vi "q2DCM (SubVI).vi"(11 "Quaternion":sgl[](array[numeric])=[0.0, 0.0, 0.0, 1.0]) -> (1 "DCM line 3":sgl[](array[numeric]), 2 "DCM line 2":sgl[](array[numeric]), 3 "DCM line 1":sgl[](array[numeric]))   [LabVIEW 2017]
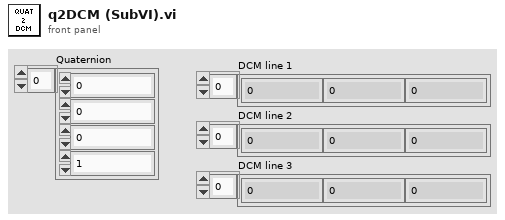
[diagram p1: front panel]
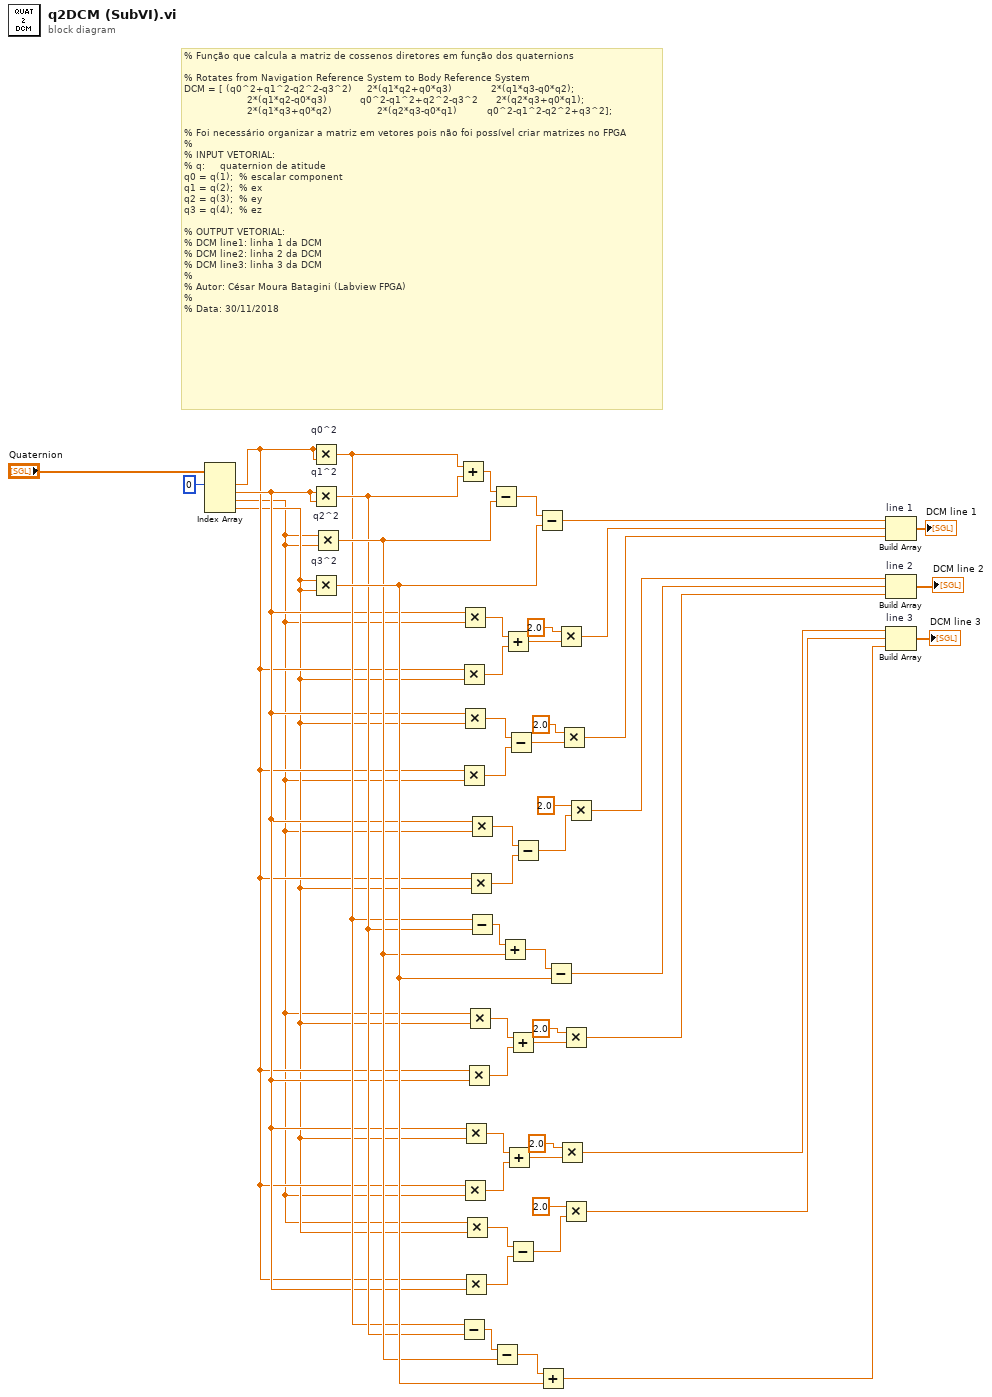
[diagram p0: block diagram]
diagram:
  # "% Função que calcula a matriz de cossenos diretores em função dos quaternions\n\n% Rotates from Navigation Reference System to Body Reference System\nDCM = [ (q0^2+q1^2-q2^2-q3^2)     2*(q1*q2+q0*q3)             2*(q1*q3-q0*q2);\n                     2*(q1*q2-q0*q3)           q0^2-q1^2+q2^2-q3^2      2*(q2*q3+q0*q1);\n                     2*(q1*q3+q0*q2)               2*(q2*q3-q0*q1)          q0^2-q1^2-q2^2+q3^2];\n\n% Foi necessário organizar a matriz em vetores pois não foi possível criar matrizes no FPGA\n%\n% INPUT VETORIAL: \n% q:     quaternion de atitude   \nq0 = q(1);  % escalar component\nq1 = q(2);  % ex\nq2 = q(3);  % ey\nq3 = q(4);  % ez\n\n% OUTPUT VETORIAL:\n% DCM line1: linha 1 da DCM\n% DCM line2: linha 2 da DCM\n% DCM line3: linha 3 da DCM\n%\n% Autor: César Moura Batagini (Labview FPGA)\n%             \n% Data: 30/11/2018"
  n1 = Index Array(array="Quaternion", index #1=0 ("index")) -> (element #1=w47:sgl, element #2=w48:sgl, element #3=w45:sgl, element #4=w46:sgl)  [unwired: 3 in]
  n2 = Multiply "q0^2"(x=w47, y=w47) -> (x*y=w49:sgl)
  n3 = Multiply "q1^2"(x=w48, y=w48) -> (x*y=w50:sgl)
  n4 = Multiply "q3^2"(x=w46, y=w46) -> (x*y=w52:sgl)
  n5 = Multiply "q2^2"(x=w45, y=w45) -> (x*y=w51:sgl)
  n6 = Add(x=w49, y=w50) -> (x+y=w14:sgl)
  n7 = Multiply(x=w47, y=w46) -> (x*y=w18:sgl)
  n8 = Multiply(x=w47, y=w45) -> (x*y=w26:sgl)
  n9 = Subtract(x=w49, y=w50) -> (x-y=w42:sgl)
  n10 = Multiply(x=w48, y=w45) -> (x*y=w17:sgl)
  n11 = Multiply(x=w48, y=w46) -> (x*y=w25:sgl)
  n12 = Multiply(x=w47, y=w45) -> (x*y=w36:sgl)
  n13 = Multiply(x=w48, y=w46) -> (x*y=w35:sgl)
  n14 = Multiply(x=w47, y=w48) -> (x*y=w40:sgl)
  n15 = Multiply(x=w45, y=w46) -> (x*y=w39:sgl)
  n16 = Multiply(x=w47, y=w48) -> (x*y=w31:sgl)
  n17 = Multiply(x=w45, y=w46) -> (x*y=w32:sgl)
  n18 = Multiply(x=w47, y=w46) -> (x*y=w21:sgl)
  n19 = Multiply(x=w48, y=w45) -> (x*y=w22:sgl)
  n20 = Subtract(x=w49, y=w50) -> (x-y=w29:sgl)
  n21 = Subtract(x=w14, y=w51) -> (x-y=w15:sgl)
  n22 = Subtract(x=w42, y=w51) -> (x-y=w43:sgl)
  n23 = Add(x=w29, y=w51) -> (x+y=w28:sgl)
  n24 = Add(x=w17, y=w18) -> (x+y=w19:sgl)
  n25 = Add(x=w35, y=w36) -> (x+y=w37:sgl)
  n26 = Subtract(x=w25, y=w26) -> (x-y=w27:sgl)
  n27 = Add(x=w32, y=w31) -> (x+y=w30:sgl)
  n28 = Subtract(x=w39, y=w40) -> (x-y=w41:sgl)
  n29 = Subtract(x=w22, y=w21) -> (x-y=w20:sgl)
  n30 = Subtract(x=w15, y=w52) -> (x-y=w10:sgl)
  n31 = Add(x=w43, y=w52) -> (x+y=w44:sgl)
  n32 = Subtract(x=w28, y=w52) -> (x-y=w5:sgl)
  n33 = Multiply(x=sgl 2.0, y=w19) -> (x*y=w9:sgl)
  n34 = Multiply(x=sgl 2.0, y=w37) -> (x*y=w2:sgl)
  n35 = Multiply(x=sgl 2.0, y=w27) -> (x*y=w8:sgl)
  n36 = Multiply(x=sgl 2.0, y=w30) -> (x*y=w4:sgl)
  n37 = Multiply(x=sgl 2.0, y=w41) -> (x*y=w1:sgl)
  n38 = Multiply(x=sgl 2.0, y=w20) -> (x*y=w6:sgl)
  n39 = Build Array "line 1"(w10, w9, w8) -> (→"DCM line 1":sgl[])
  n40 = Build Array "line 2"(w6, w5, w4) -> (→"DCM line 2":sgl[])
  n41 = Build Array "line 3"(w2, w1, w44) -> (→"DCM line 3":sgl[])
